vi "Instrument_Write&Read.vi"(7 "Read?":bool=TRUE, 8 "Error In":errorcluster, 9 "CMD":string, 10 "wait ms":i32=100, 11 "PORT":string) -> (0 "Error Out":errorcluster, 2 "read buffer":string)   [LabVIEW 2013]
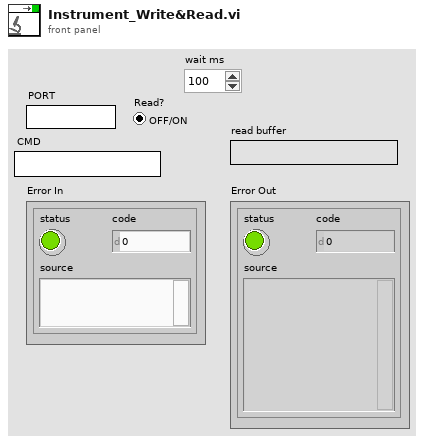
[diagram p1: front panel]
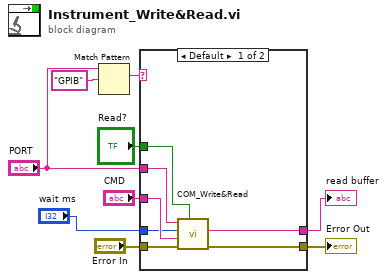
[diagram p0: block diagram]
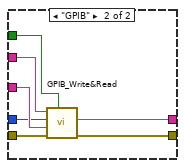
[diagram p2: hidden frame]
diagram:
  n1 = Match Pattern(string="PORT", regular expression="GPIB") -> (match substring=w8:string)  [unwired: 1 in, 3 out]
  n2 = case shown="Default" w8 {
    tunnel: "PORT" -> [w16 w23]
    tunnel: "CMD" -> [w11 w22]
    tunnel: [w15 w21] -> w4
    tunnel: "Read?" -> [w14 w20]
    tunnel: "Error In" -> [w13 w19]
    tunnel: [w12 w18] -> w2
    tunnel: "wait ms" -> [w10 w17]
    frame Default {
      n3 = call "COM_Write&Read.vi"("Read?"=w14, "error in (no error)"=w13, "String"=w11, "wait ms"=w10, "VISA Refnum in"=w16) -> ("error out"=w12:errorcluster, "read buffer"=w15:string)  [unwired: 4 in, 1 out]
    }
    frame "GPIB" {
      n4 = call "GPIB_Write&Read.vi"("Read?"=w20, "error in (no error)"=w19, "String"=w22, "wait ms"=w17, "GPIB Addr"=w23) -> ("error out"=w18:errorcluster, "read buffer"=w21:string)  [unwired: 5 in]
    }
  }
  "read buffer" <- w4
  "Error Out" <- w2
